vi "MultiAxisControl.vi"() -> ()   [LabVIEW 2026]
uses:
  Utility/AxisControl.ctl
  Parameters/GetAxisParameterString.vi
  Parameters/GetAxisParameterDouble.vi
  Motion/AbortSingle.vi
  Motion/MoveIncSingle.vi
  Motion/FreerunSingle.vi
  Motion/EnableSingle.vi
  Motion/DisableSingle.vi
  Motion/FaultAckSingle.vi
  Motion/HomeSingle.vi
panel:
  in  "Disconnect?":bool
  in  "Show First":i32=2 caption="Axes" min=0 max=32
  out "Status":string
  in  "StopProgram":bool caption="Stop"
  out "do stop":bool
  in  "stop":bool
  out "Error":string
  in  "Init":bool=TRUE
  in  "Abort Motion":bool
  in  "Reset Controller":bool
  in  "In Task:":i32(ring)=1 items=["TLibrary", "T01", "T02", "T03", "T04", "T05", "T06", "T07", "T08", "T09", "T10", "T11", "T12", "T13", "T14", "T15", "T16", "T17", "T18", "T19", "T20", "T21", "T22", "T23", "T24", "T25", "T26", "T27", "T28", "T29", "T30", "T31"]
  in  "ExecuteProgram":bool caption="Execute"
  in  "Program:":path
  in  "Axes":T1[](array[typedef])
  in  "Status":string
  in  "Execute":bool
  in  "Command:":string
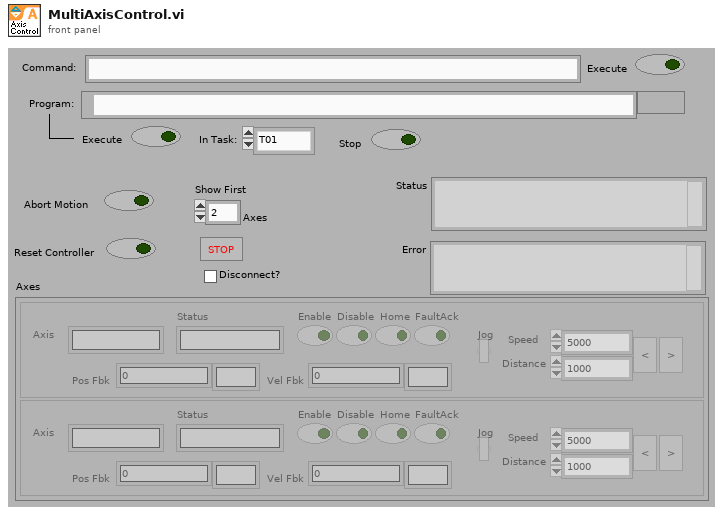
[diagram p1: front panel]
types:
  T1 = typedef "AxisControl.ctl" = cluster{"Axis":string, "Enable":bool, "Disable":bool, "Home":bool, "FaultAck":bool, "Jog":bool, "Speed":dbl, "Distance":dbl, "Jog Left":bool, "Jog Right":bool, "Status":string, "Pos Fbk":dbl, "Vel Fbk":dbl, "Pos Units":string, "Vel Units":string}
  T2 = cluster{"new reference":refnum<k24>, "Event Callback":refnum<k27>, "ControllerDiagPacket":refnum<user-event>, "Event Registration Refnum":refnum<event-registration>}
  T3 = enum32{"invalid app kind", "Development System", "Run Time System", "Student Edition", "Embedded LabVIEW", "Evaluation", "Custom"}
  T4 = cluster{"Axis":string, "Enable":bool, "Disable":bool, "Home":bool, "FaultAck":bool, "Jog":bool, "Speed":dbl, "Distance":dbl, "Jog Left":bool, "Jog Right":bool, "Status":string, "Pos Fbk":dbl, "Vel Fbk":dbl, "Pos Units":string, "Vel Units":string}
  T5 = typedef "AxisDiagPacket.ctl" = cluster{"Axis Name":string, "Analog Input 0":dbl, "Analog Input 1":dbl, "Axis Fault (num)":i32, "Axis Fault (str)":string, "Axis Fault (bits)":cluster{"AmplifierFault":bool, "AmplifierTemperatureFault":bool, "CcwEndOfTravelLimitFault":bool, "CcwSoftwareLimitFault":bool, "CommunicationLostFault":bool, "CwEndOfTravelLimitFault":bool, "CwSoftwareLimitFault":bool, "EmergencyStopFault":bool, "EncoderFault":bool, "ExternalFault":bool, "FeedbackScalingFault":bool, "GantryMisalignFault ":bool, "HallSensorFault":bool, "InPositionTimeoutFault":bool, "MarkerSearchFault":bool, "MaxVelocityCommandFault":bool, "MissedInterruptFault":bool, "MotorTemperatureFault":bool, "None":bool, "OverCurrentFault":bool, "PositionErrorFault":bool, "PositionFeedbackFault":bool, "PowerSupplyFault":bool, "ProbeInputFault":bool, "SafeZoneFault":bool, "VelocityErrorFault":bool, "VelocityFeedbackFault":bool, "VoltageClampFault":bool, "InternalFault":bool}, "Axis Status (num)":i32, "Axis Status (str)":string, "Axis Status (bits)":cluster{"BacklashActive":bool, "CalibrationEnabled1D":bool, "CalibrationEnabled2D":bool, "CommandValid":bool, "DriveAbortPending":bool, "DrivePending":bool, "Enabling":bool, "GainMappingEnabled":bool, "GantryAligned":bool, "GantryRealigning":bool, "Homed":bool, "Homing":bool, "IFOVEnabled":bool, "JogGenerating":bool, "Jogging":bool, "JoystickControl":bool, "MasterSlaveControl":bool, "MotionBlocked":bool, "MotionClamped":bool, "MoveDone":bool, "None":bool, "NotVirtual":bool, "Profiling":bool, "Stability0":bool, "Stability1":bool, "TrajectoryFiltering":bool, "WaitDone":bool}, "Current Command":sgl, "Current Error":sgl, "Current Feedback":sgl, "Digital Inputs":i32, "Digital Outputs":i32, "Drive Status":i32, "Drive Status (str)":string, "Drive Status (bits)":cluster{"AccelerationPhase":bool, "AutofocusActive":bool, "BrakeOutput":bool, "CcwEndOfTravelLimitInput":bool, "CosineEncoderError":bool, "CurrentClamp":bool, "CwEndOfTravelLimitInput":bool, "DecelerationPhase":bool, "DualLoopActive":bool, "EmergencyStopInput":bool, "Enabled":bool, "EncoderClipping":bool, "GalvoCalibrationEnabled":bool, "GalvoPowerCorrection":bool, "HallAInput":bool, "HallBInput":bool, "HallCInput":bool, "HighResolutionMode":bool, "HomeLimitInput":bool, "InPosition":bool, "InPosition2":bool, "MarkerInput":bool, "MarkerLatch":bool, "MoveActive":bool, "NoMotorSupply":bool, "None":bool, "PowerLimiting":bool, "ProgrammingFlash":bool, "ProgrammingMXH":bool, "PSOHaltLatch":bool, "ServoControl":bool, "SineEncoderError":bool}, "Position Feedback Auxiliary":dbl, "Position Command":dbl, "Position Error":dbl, "Position Feedback":dbl, "Program Position Command":dbl, "Program Position Error":dbl, "Program Position Feedback":dbl, "Velocity Command":dbl, "Velocity Error":dbl, "Velocity Feedback":dbl}
  T6 = cluster{"Axis":string, "Enable":bool, "Disable":bool, "Home":bool, "FaultAck":bool, "Jog":bool, "Speed":dbl, "Distance":dbl, "Jog Left":bool, "Jog Right":bool, "Status":string, "Pos Fbk":dbl, "Vel Fbk":dbl, "Pos Units":string, "Vel Units":string}[]
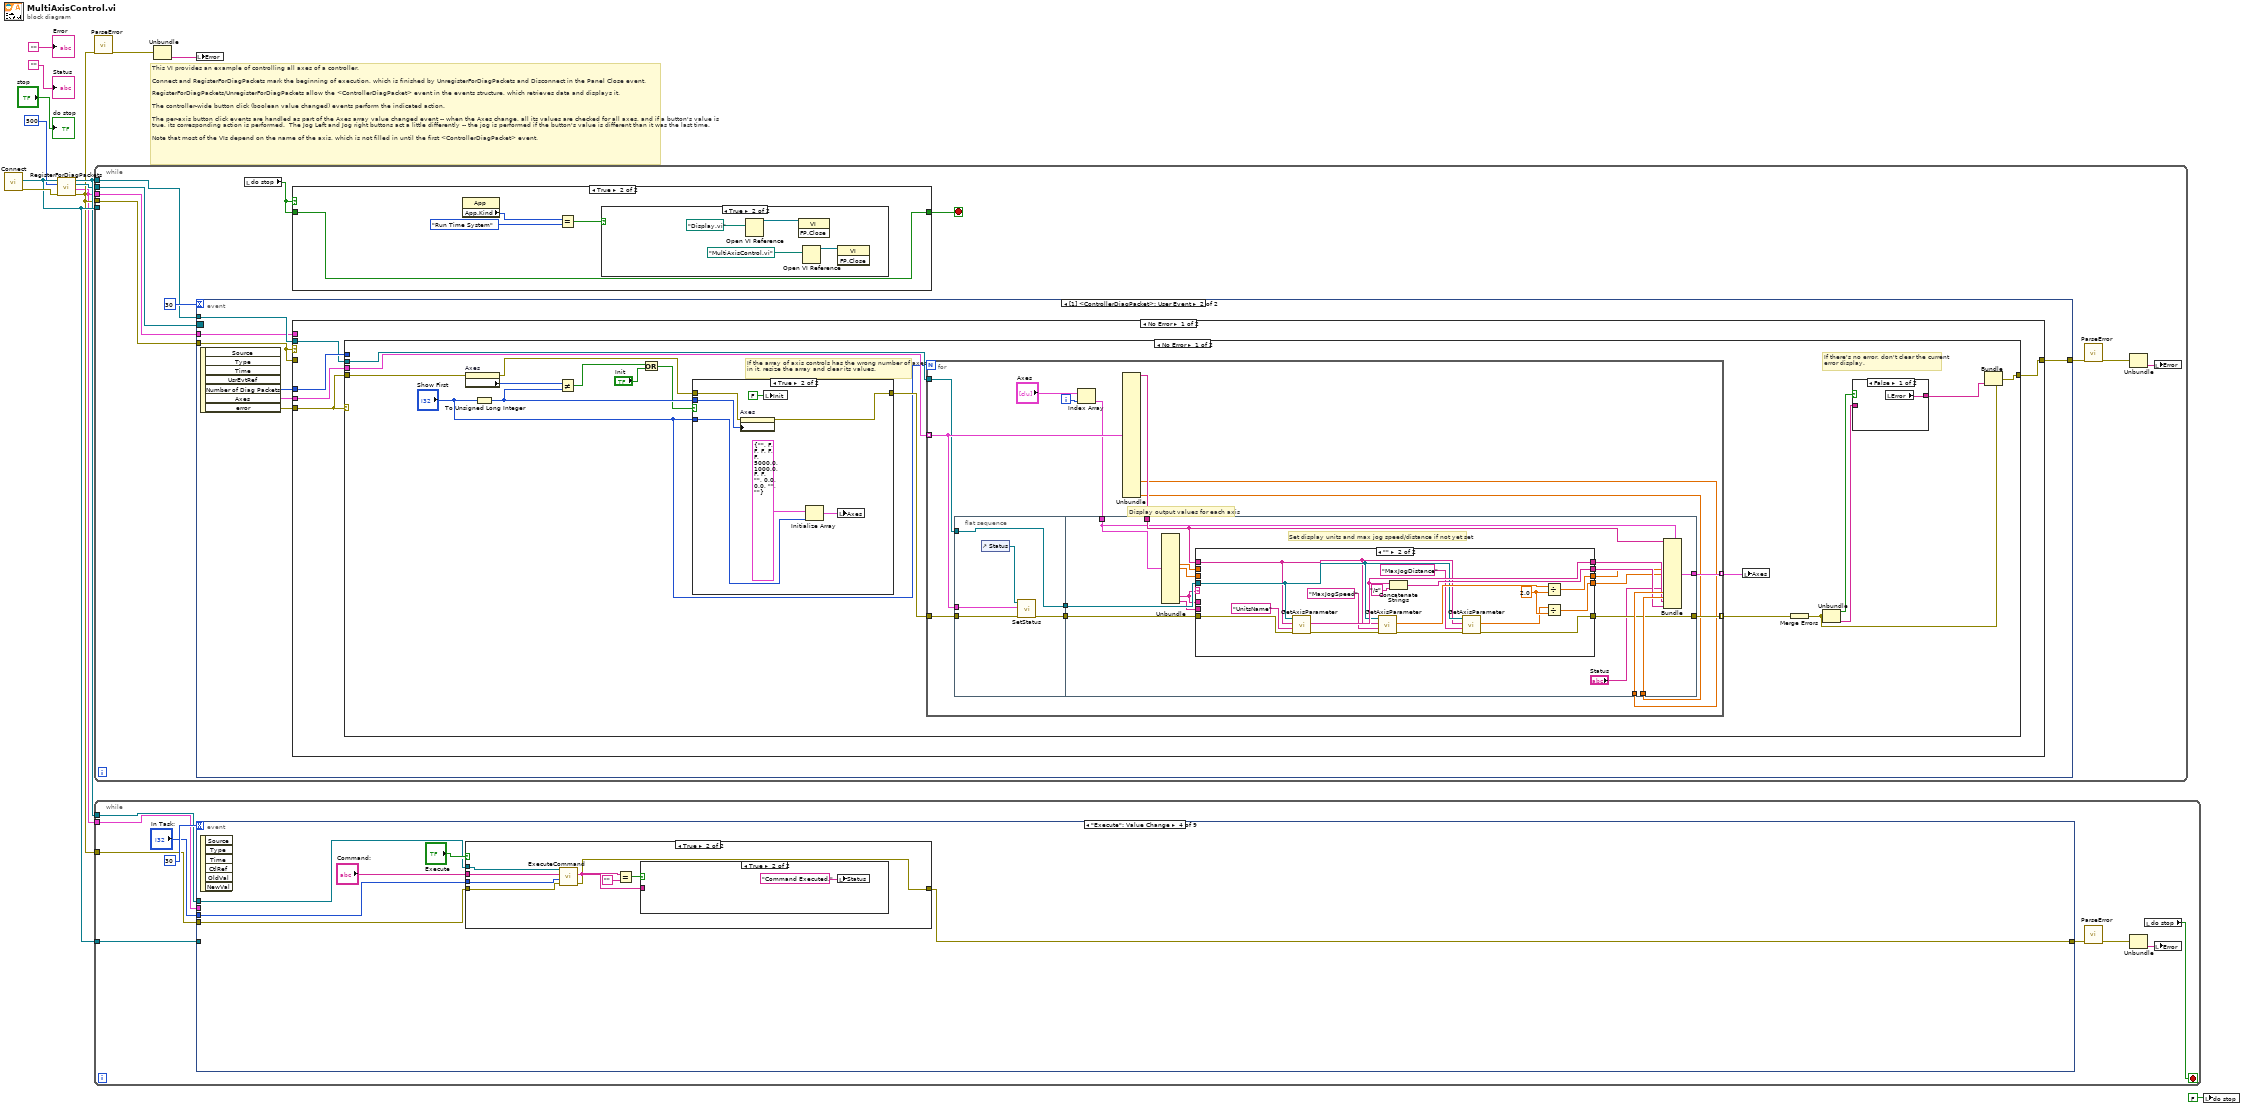
[diagram p0: block diagram]
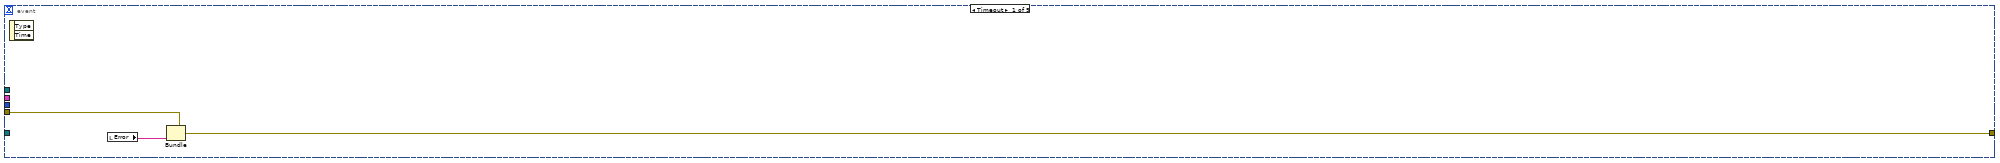
[diagram p2: hidden frame]
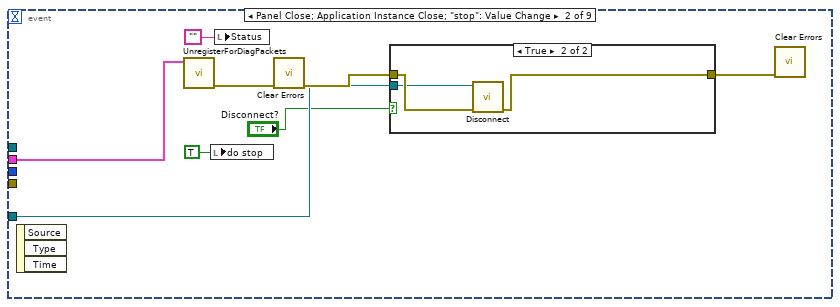
[diagram p3: hidden frame]
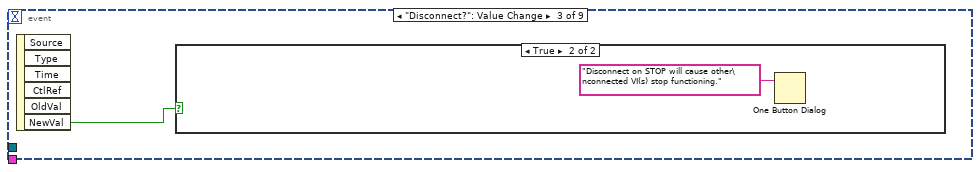
[diagram p5: hidden frame]
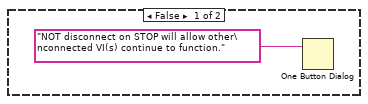
[diagram p6: hidden frame]
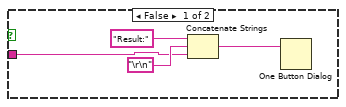
[diagram p8: hidden frame]
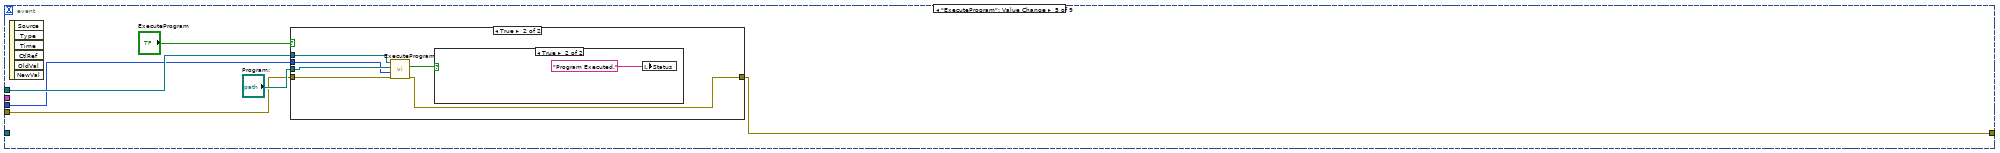
[diagram p9: hidden frame]
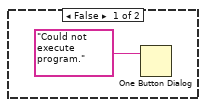
[diagram p11: hidden frame]
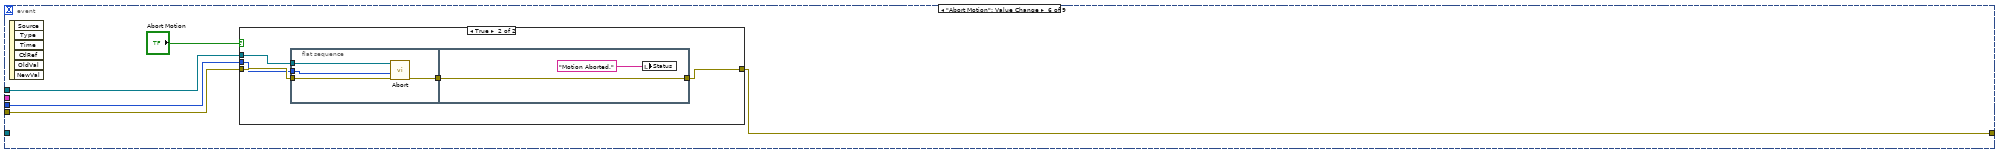
[diagram p12: hidden frame]
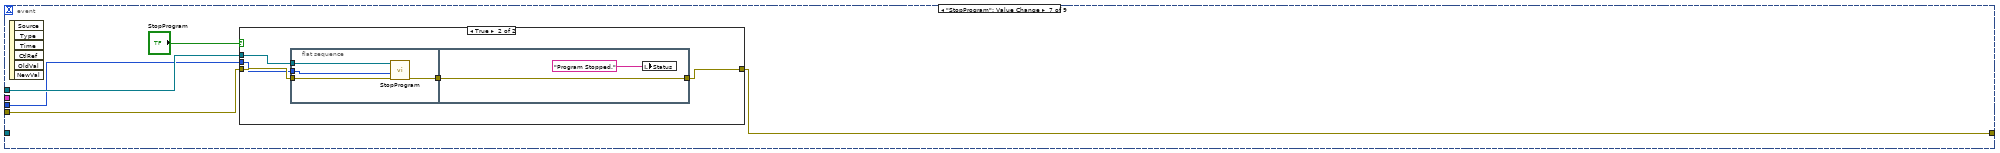
[diagram p14: hidden frame]
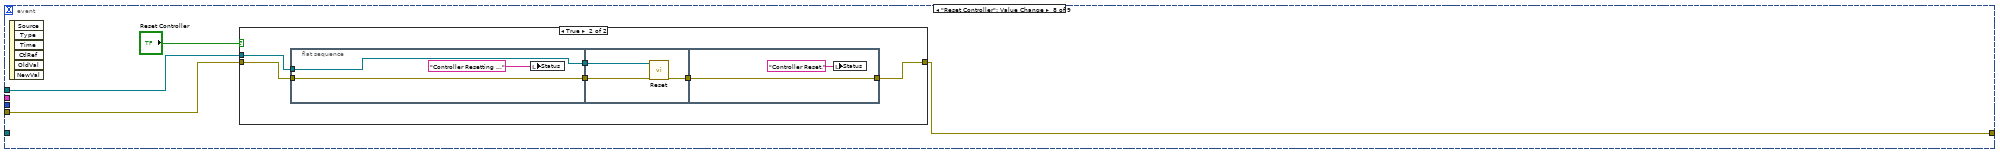
[diagram p16: hidden frame]
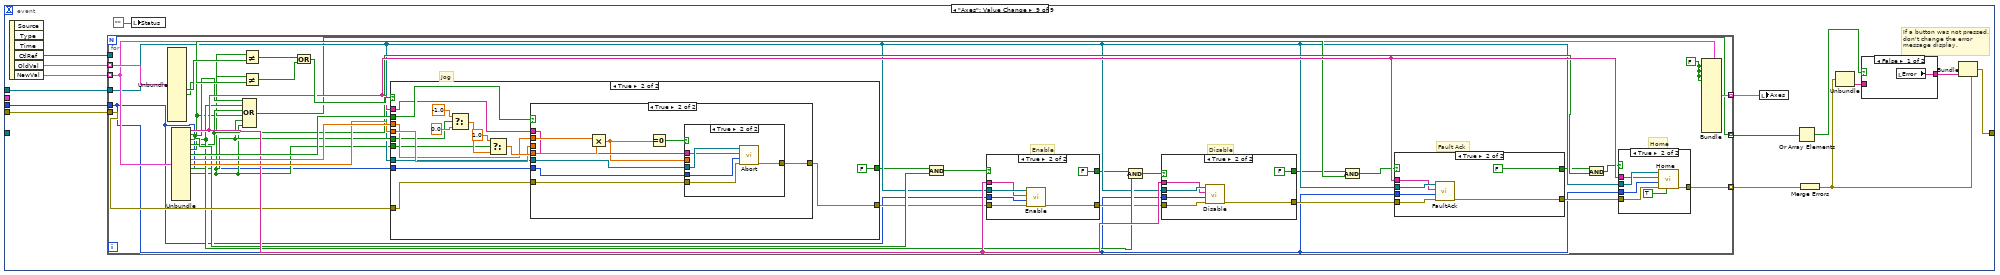
[diagram p18: hidden frame]
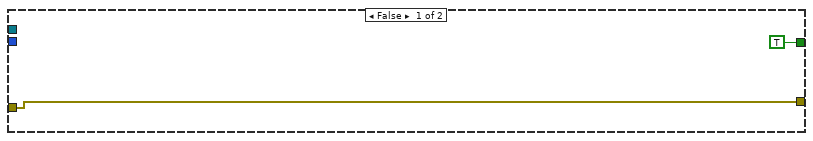
[diagram p20: hidden frame]
diagram:
  # "This VI provides an example of controlling all axes of a controller. \n\nConnect and RegisterForDiagPackets mark the beginning of execution, which is finished by UnregisterForDiagPackets and Disconnect in the Panel Close event.\n\nRegisterForDiagPackets/UnregisterForDiagPackets allow the <ControllerDiagPacket> event in the events structure, which retrieves data and displays it.\n\nThe controller-wide button click (boolean value changed) events perform the indicated action.\n\nThe per-axis button click events are handled as part of the Axes array value changed event -- when the Axes change, all its values are checked for all axes, and if a button's value is true, its corresponding action is performed.  The Jog Left and Jog right buttons act a little differently -- the jog is performed if the button's value is different than it was the last time.\n\nNote that most of the VIs depend on the name of the axis, which is not filled in until the first <ControllerDiagPacket> event."
  n1 = call "Connect.vi"() -> ("error out"=w7:errorcluster, "controller"=w6:refnum<k24>)  [unwired: 10 in]
  n2 = call "RegisterForDiagPackets.vi"("error in (no error)"=w7, "refresh interval (default)"=500, "Controller in"=w6) -> ("error out"=w3:errorcluster, "Event Metadata"=w2:T2, "Event Registration Refnum"=w4:refnum<event-registration>, "Controller out"=w5:refnum<k24>)  [unwired: 4 in]
  n3 = call "ParseError.vi"("error in (no error)"=w3) -> ("error out"=w11:errorcluster)  [unwired: 10 in]
  n4 = while {
    tunnel: w4 -> [w20]
    tunnel: w5 -> [w18]
    tunnel: w6 -> [_]
    tunnel: w3 -> [w17]
    tunnel: w2 -> [w16]
    stop <- w15 stop-if-true
    n5 = event shown="[1] <ControllerDiagPacket>: User Event" {
      selector: w20 -> [_ _]
      dyn-events: _ -> [_ _]
      timeout: 30 -> [_ _]
      tunnel: [w33 w42] -> w19
      tunnel: w18 -> [_ w41]
      tunnel: w17 -> [w35 w40]
      tunnel: w16 -> [_ w36]
      event Timeout {
        n6 = event-data() -> ()  [unwired: 1 in, 2 out]
        n7 = local read "Error"() -> (w34:string)
        n8 = Bundle(cluster=w35, "source"=w34) -> (w33:errorcluster)  [unwired: 2 in]
      }
      event User Event {
        n9 = event-data() -> ("Number of Diag Packets"=w39:i32, "Axes"=w38:T5[], "error"=w37:errorcluster)  [unwired: 1 in, 4 out]
        n10 = case shown="No Error" w40 {
          tunnel: w38 -> [w47 _]
          tunnel: [w46 w134] -> w42
          tunnel: w39 -> [w45 _]
          tunnel: w37 -> [w44 _]
          tunnel: w40 -> [_ w134]
          tunnel: w41 -> [w43 _]
          tunnel: w36 -> [_ _]
          frame No Error {
            n11 = case shown="No Error" w44 {
              tunnel: w47 -> [w65 _]
              tunnel: [w55 w133] -> w46
              tunnel: w44 -> [w51 w133]
              tunnel: w45 -> [_ _]
              tunnel: w43 -> [w49 _]
              frame No Error {
                # "If there's no error, don't clear the current error display."
                # "If the array of axis controls has the wrong number of axes in it, resize the array and clear its values."
                n12 = property on="Axes" class="Arr (strict)"(error in=w51) -> (error out=w50:errorcluster, "Number of Rows"=w61:u32)  [unwired: 1 in, 1 out]
                n13 = To Unsigned Long Integer(number="Show First") -> (unsigned 32bit integer=w60:u32)
                n14 = Not Equal?(x=w61, y=w60) -> (x != y?=w59:bool)
                n15 = Or(x=w59, y="Init") -> (x .or. y?=w58:bool)
                n16 = case shown="True" w58 {
                  tunnel: w50 -> [w125 w132]
                  tunnel: [w125 w131] -> w64
                  tunnel: w60 -> [_ w127]
                  tunnel: "Show First" -> [_ w128]
                  frame False {
                  }
                  frame True {
                    n17 = property on="Axes" class="Arr (strict)"(error in=w132, "Number of Rows"=w127) -> (error out=w131:errorcluster)  [unwired: 1 in, 1 out]
                    n18 = local write "Init"(FALSE ("Init")) -> ()
                    n19 = Initialize Array(T4 {"Axis"="", "Enable"=FALSE, "Disable"=FALSE, "Home"=FALSE, "FaultAck"=FALSE, "Jog"=FALSE, "Speed"=5000.0, "Distance"=1000.0, "Jog Left"=FALSE, "Jog Right"=FALSE, "Status"="", "Pos Fbk"=0.0, "Vel Fbk"=0.0, "Pos Units"="", "Vel Units"=""} ("Axis"), w128) -> (w130:T6)
                    n20 = local write "Axes"(w130) -> ()
                  }
                }
                n21 = for {
                  N: "Show First" -> [_]
                  tunnel: w64 -> [w79]
                  tunnel: w65 -> [w80] mode=indexing
                  tunnel: [w78] -> w63 mode=indexing
                  tunnel: [w73] -> w62 mode=indexing
                  tunnel: w49 -> [w71]
                  i -> [w74]
                  # "Display output values for each axis"
                  n22 = flat-sequence {
                    tunnel: w80 -> [w84]
                    tunnel: w79 -> [w83]
                    tunnel: [w82] -> w72
                    tunnel: w71 -> [w81]
                    tunnel: [w81] -> w70
                    tunnel: w75 -> [w95]
                    tunnel: w77 -> [w97]
                    tunnel: w69 -> [w101]
                    tunnel: w68 -> [w100]
                    tunnel: w72 -> [w98]
                    tunnel: w70 -> [w96]
                    tunnel: [w102] -> w78
                    tunnel: [w99] -> w73
                    frame #0 {
                      n23 = control-ref of="Status"() -> (w85:refnum<vi>)
                      n24 = call "SetStatus.vi"("error in (no error)"=w83, "AxisDiagPacket"=w84, "Status string"=w85) -> ("error out"=w82:errorcluster)  [unwired: 8 in]
                    }
                    frame #1 {
                      # "Set display units and max jog speed/distance if not yet set"
                      n25 = Unbundle(w95) -> ("Speed"=w90:dbl, "Distance"=w89:dbl, "Pos Units"=w94:string, "Vel Units"=w93:string)  [unwired: 11 out]
                      n26 = case shown="\"\"" w94 {
                        tunnel: w96 -> [_ w109]
                        tunnel: [w107 w112] -> w99
                        tunnel: w98 -> [w107 w122]
                        tunnel: w97 -> [_ w108]
                        tunnel: w94 -> [w105 _]
                        tunnel: w93 -> [w106 _]
                        tunnel: [w106 w121] -> w92
                        tunnel: [w105 w120] -> w91
                        tunnel: w90 -> [w104 _]
                        tunnel: w89 -> [w103 _]
                        tunnel: [w104 w111] -> w88
                        tunnel: [w103 w110] -> w87
                        frame Default {
                        }
                        frame "" {
                          w119 = 2.0 ("y")
                          n27 = call-poly "GetAxisParameter.vi"("error in (no error)"=w122, "Parameter Name"="UnitsName" ("parameter name"), "axis name"=w108, "controller in"=w109) -> ("error out"=w113:errorcluster, "value"=w120:string)  [unwired: 5 in, 1 out]
                          n28 = call-poly "GetAxisParameter.vi"("error in (no error)"=w113, "Parameter Name"="MaxJogSpeed" ("parameter name"), "axis name"=w108, "controller in"=w109) -> ("error out"=w114:errorcluster, "value"=w117:dbl)  [unwired: 5 in, 1 out]
                          n29 = Concatenate Strings(w120, "/s" ("string")) -> (w121:string)
                          n30 = call-poly "GetAxisParameter.vi"("error in (no error)"=w114, "Parameter Name"="MaxJogDistance" ("parameter name"), "axis name"=w108, "controller in"=w109) -> ("error out"=w112:errorcluster, "value"=w118:dbl)  [unwired: 5 in, 1 out]
                          n31 = Divide(x=w117, y=w119) -> (x/y=w111:dbl)
                          n32 = Divide(x=w118, y=w119) -> (x/y=w110:dbl)
                        }
                      }
                      n33 = Bundle(cluster=w95, "Axis"=w97, "Speed"=w88, "Distance"=w87, "Status"="Status", "Pos Fbk"=w101, "Vel Fbk"=w100, "Pos Units"=w91, "Vel Units"=w92) -> (w102:T1)  [unwired: 7 in]
                    }
                  }
                  n34 = Index Array(array="Axes", index=w74) -> (element=w75:T1)
                  n35 = Unbundle(w80) -> ("Axis Name"=w77:string, "Program Position Feedback"=w69:dbl, "Velocity Feedback"=w68:dbl)  [unwired: 24 out]
                }
                n36 = local write "Axes"(w63) -> ()
                n37 = Merge Errors(w62) -> (w56:errorcluster)
                n38 = Unbundle(w56) -> ("status"=w54:bool, "source"=w53:string)  [unwired: 1 out]
                n39 = case shown="False" w54 {
                  tunnel: w53 -> [_ w67]
                  tunnel: [w66 w67] -> w52
                  frame False {
                    n40 = local read "Error"() -> (w66:string)
                  }
                  frame True {
                  }
                }
                n41 = Bundle(cluster=w56, "source"=w52) -> (w55:errorcluster)  [unwired: 2 in]
              }
              frame Error {
              }
            }
          }
          frame Error {
          }
        }
      }
    }
    n42 = local read "do stop"() -> (w14:bool)
    n43 = case shown="True" w14 {
      tunnel: w14 -> [w24 w28]
      tunnel: [w24 w28] -> w15
      frame False {
      }
      frame True {
        n44 = property class="App"() -> ("App.Kind"=w27:T3)  [unwired: 2 in, 2 out]
        n45 = Equal?(x=w27, y=T3."Run Time System" ("Application:Kind")) -> (x = y?=w25:bool)
        n46 = case shown="True" w25 {
          frame False {
          }
          frame True {
            n47 = Open VI Reference(vi path=path "Display.vi") -> (vi reference=w29:refnum<vi>)  [unwired: 5 in, 1 out]
            n48 = invoke class="VI" method="FP.Close"(reference=w29) -> ()  [unwired: 2 in, 3 out]
            n49 = Open VI Reference(vi path=path "MultiAxisControl.vi") -> (vi reference=w31:refnum<vi>)  [unwired: 5 in, 1 out]
            n50 = invoke class="VI" method="FP.Close"(reference=w31) -> ()  [unwired: 2 in, 3 out]
          }
        }
      }
    }
    n51 = call "ParseError.vi"("error in (no error)"=w19) -> ("error out"=w22:errorcluster)  [unwired: 10 in]
    n52 = Unbundle(w22) -> ("source"=w23:string)  [unwired: 2 out]
    n53 = local write "Error"(w23) -> ()
  }
  n54 = while {
    tunnel: w6 -> [w140]
    tunnel: w5 -> [w139]
    tunnel: w3 -> [w138]
    tunnel: w2 -> [w135]
    stop <- w137 stop-if-true
    n55 = event shown="[3] \"Execute\": Value Change" {
      selector: _ -> [_ _ _ _ _ _ _ _ _]
      dyn-events: _ -> [_ _ _ _ _ _ _ _ _]
      timeout: 30 -> [_ _ _ _ _ _ _ _ _]
      tunnel: w139 -> [_ _ _ w167 w187 w201 w216 w234 w263]
      tunnel: w138 -> [w147 _ _ w166 w185 w202 w218 w233 w262]
      tunnel: [w146 _ _ w164 w184 w199 w217 w232 w257] -> w142
      tunnel: w140 -> [_ w154 _ _ _ _ _ _ _]
      tunnel: "In Task:" -> [_ _ _ w163 w183 w198 w215 _ w251]
      tunnel: w135 -> [_ w148 _ _ _ _ _ _ _]
      event Timeout {
        n56 = event-data() -> ()  [unwired: 1 in, 2 out]
        n57 = local read "Error"() -> (w145:string)
        n58 = Bundle(cluster=w147, "source"=w145) -> (w146:errorcluster)  [unwired: 2 in]
      }
      event Panel Close; Application Instance Close; "stop": Value Change {
        n59 = event-data() -> ()  [unwired: 1 in, 3 out]
        n60 = call "UnregisterForDiagPackets.vi"("Event Metadata"=w148) -> ("error out"=w149:errorcluster)  [unwired: 9 in]
        n61 = local write "do stop"(TRUE) -> ()
        n62 = local write "Status"("") -> ()
        n63 = call <vilib>:"Clear Errors.vi"("error in (no error)"=w149) -> ("error out"=w155:errorcluster)  [unwired: 5 in, 1 out]
        n64 = case shown="True" "Disconnect?" {
          tunnel: w155 -> [w156 w159]
          tunnel: w154 -> [_ w158]
          tunnel: [w156 w157] -> w153
          frame False {
          }
          frame True {
            n65 = call "Disconnect.vi"("error in (no error)"=w159, "controller"=w158) -> ("error out"=w157:errorcluster)  [unwired: 9 in]
          }
        }
        n66 = call <vilib>:"Clear Errors.vi"("error in (no error)"=w153) -> ()  [unwired: 5 in, 2 out]
      }
      event "Disconnect?": Value Change {
        n67 = event-data() -> ("NewVal"=w160:bool)  [unwired: 1 in, 5 out]
        n68 = case shown="True" w160 {
          frame False {
            n69 = One Button Dialog(message="NOT disconnect on STOP will allow other\nconnected VI(s) continue to function.") -> ()  [unwired: 1 in, 1 out]
          }
          frame True {
            n70 = One Button Dialog(message="Disconnect on STOP will cause other\nconnected VI(s) stop functioning.") -> ()  [unwired: 1 in, 1 out]
          }
        }
      }
      event "Execute": Value Change {
        n71 = event-data() -> ()  [unwired: 1 in, 6 out]
        n72 = case shown="True" "Execute" {
          tunnel: w167 -> [_ w177]
          tunnel: w166 -> [w169 w175]
          tunnel: "Command:" -> [_ w176]
          tunnel: [w169 w171] -> w164
          tunnel: w163 -> [_ w170]
          frame False {
          }
          frame True {
            n73 = call "ExecuteCommand.vi"("error in (no error)"=w175, "taskId"=w170, "Command Code"=w176, "controller in"=w177) -> ("error out"=w171:errorcluster, "return value"=w172:string)  [unwired: 5 in, 1 out]
            n74 = Equal?(x=w172, y="") -> (x = y?=w173:bool)
            n75 = case shown="True" w173 {
              tunnel: w172 -> [w178 _]
              frame False {
                n76 = Concatenate Strings("Result:", "\r\n", w178) -> (w181:string)
                n77 = One Button Dialog(message=w181) -> ()  [unwired: 1 in, 1 out]
              }
              frame True {
                n78 = local write "Status"("Command Executed." ("Status")) -> ()
              }
            }
          }
        }
      }
      event "ExecuteProgram": Value Change {
        n79 = event-data() -> ()  [unwired: 1 in, 6 out]
        n80 = case shown="True" "ExecuteProgram" {
          tunnel: w187 -> [_ w195]
          tunnel: w185 -> [w189 w193]
          tunnel: "Program:" -> [_ w194]
          tunnel: w183 -> [_ w191]
          tunnel: [w189 w190] -> w184
          frame False {
          }
          frame True {
            n81 = call "ExecuteProgram.vi"("error in (no error)"=w193, "taskId"=w191, "program name and path"=w194, "controller in"=w195) -> ("error out"=w190:errorcluster, "success"=w192:bool)  [unwired: 5 in, 1 out]
            n82 = case shown="True" w192 {
              frame False {
                n83 = One Button Dialog(message="Could not execute program.") -> ()  [unwired: 1 in, 1 out]
              }
              frame True {
                n84 = local write "Status"("Program Executed." ("Status")) -> ()
              }
            }
          }
        }
      }
      event "Abort Motion": Value Change {
        n85 = event-data() -> ()  [unwired: 1 in, 6 out]
        n86 = case shown="True" "Abort Motion" {
          tunnel: w201 -> [_ w208]
          tunnel: w202 -> [w203 w207]
          tunnel: [w203 w206] -> w199
          tunnel: w198 -> [_ w204]
          frame False {
          }
          frame True {
            n87 = flat-sequence {
              tunnel: w208 -> [w212]
              tunnel: w207 -> [w211]
              tunnel: [w210] -> w205
              tunnel: w204 -> [w209]
              tunnel: [w214] -> w206
              tunnel: w205 -> [w214]
              frame #0 {
                n88 = call-poly "Abort.vi"("error in (no error)"=w211, "taskId"=w209, "controller in"=w212) -> ("error out"=w210:errorcluster)  [unwired: 7 in, 1 out]
              }
              frame #1 {
                n89 = local write "Status"("Motion Aborted." ("Status")) -> ()
              }
            }
          }
        }
      }
      event "StopProgram": Value Change {
        n90 = event-data() -> ()  [unwired: 1 in, 6 out]
        n91 = case shown="True" "StopProgram" {
          tunnel: w218 -> [w220 w225]
          tunnel: [w220 w224] -> w217
          tunnel: w216 -> [_ w223]
          tunnel: w215 -> [_ w221]
          frame False {
          }
          frame True {
            n92 = flat-sequence {
              tunnel: w225 -> [w229]
              tunnel: w223 -> [w227]
              tunnel: [w228] -> w222
              tunnel: w221 -> [w226]
              tunnel: [w231] -> w224
              tunnel: w222 -> [w231]
              frame #0 {
                n93 = call "StopProgram.vi"("error in (no error)"=w229, "taskId"=w226, "controller in"=w227) -> ("error out"=w228:errorcluster)  [unwired: 7 in, 1 out]
              }
              frame #1 {
                n94 = local write "Status"("Program Stopped." ("Status")) -> ()
              }
            }
          }
        }
      }
      event "Reset Controller": Value Change {
        n95 = event-data() -> ()  [unwired: 1 in, 6 out]
        n96 = case shown="True" "Reset Controller" {
          tunnel: w234 -> [_ w242]
          tunnel: w233 -> [w236 w241]
          tunnel: [w236 w240] -> w232
          frame False {
          }
          frame True {
            n97 = flat-sequence {
              tunnel: w241 -> [w244]
              tunnel: w242 -> [w245]
              tunnel: [w245] -> w239
              tunnel: [w244] -> w238
              tunnel: w239 -> [w248]
              tunnel: w238 -> [w247]
              tunnel: [w246] -> w237
              tunnel: [w250] -> w240
              tunnel: w237 -> [w250]
              frame #0 {
                n98 = local write "Status"("Controller Resetting ..." ("Errors")) -> ()
              }
              frame #1 {
                n99 = call "Reset.vi"("error in (no error)"=w247, "controller in"=w248) -> ("error out"=w246:errorcluster)  [unwired: 8 in, 1 out]
              }
              frame #2 {
                n100 = local write "Status"("Controller Reset." ("Status")) -> ()
              }
            }
          }
        }
      }
      event "Axes": Value Change {
        # "If a button was not pressed, don't change the error message display."
        n101 = event-data() -> ("CtlRef"=w264:refnum<vi>, "OldVal"=w261:T1[], "NewVal"=w265:T1[])  [unwired: 1 in, 3 out]
        n102 = for {
          tunnel: w265 -> [w287] mode=indexing
          tunnel: w264 -> [_]
          tunnel: w263 -> [w285]
          tunnel: w262 -> [w293]
          tunnel: w261 -> [w300] mode=indexing
          tunnel: [w274] -> w260 mode=indexing
          tunnel: [w270] -> w259 mode=indexing
          tunnel: [w288] -> w254 mode=indexing
          tunnel: w251 -> [w268]
          w269 = FALSE
          # "Jog"
          # "Fault Ack"
          # "Home"
          # "Disable"
          # "Enable"
          n103 = Unbundle(w300) -> ("Jog Left"=w296:bool, "Jog Right"=w295:bool)  [unwired: 13 out]
          n104 = Unbundle(w287) -> ("Axis"=w294:string, "Enable"=w292:bool, "Disable"=w291:bool, "Home"=w290:bool, "FaultAck"=w289:bool, "Jog"=w301:bool, "Speed"=w303:dbl, "Distance"=w302:dbl, "Jog Left"=w286:bool, "Jog Right"=w275:bool)  [unwired: 5 out]
          n105 = Compound Arithmetic op=OR(w292, w291, w290, w289, w286, w275) -> (w270:bool)
          n106 = Not Equal?(x=w275, y=w296) -> (x != y?=w298:bool)
          n107 = Not Equal?(x=w286, y=w295) -> (x != y?=w297:bool)
          n108 = Or(x=w298, y=w297) -> (x .or. y?=w299:bool)
          n109 = case shown="True" w299 {
            tunnel: w301 -> [_ w316]
            tunnel: w303 -> [_ w314]
            tunnel: w302 -> [_ w315]
            tunnel: w275 -> [_ w310]
            tunnel: w286 -> [_ w309]
            tunnel: w285 -> [_ w313]
            tunnel: w294 -> [_ w312]
            tunnel: w293 -> [w305 w311]
            tunnel: [w305 w308] -> w278
            tunnel: [TRUE FALSE] -> w283
            tunnel: w268 -> [_ w306]
            frame False {
            }
            frame True {
              n110 = Select(t=-1.0, s=w309, f=0.0) -> (s? t:f=w321:dbl)
              n111 = Select(t=1.0, s=w310, f=w321) -> (s? t:f=w317:dbl)
              n112 = case shown="True" w316 {
                tunnel: w314 -> [w325 w339]
                tunnel: w315 -> [w330 _]
                tunnel: w317 -> [w329 w338]
                tunnel: w311 -> [w328 w337]
                tunnel: w312 -> [w324 w336]
                tunnel: w313 -> [w323 w335]
                tunnel: [w327 w334] -> w308
                tunnel: w306 -> [w322 w333]
                frame False {
                  n113 = Multiply(x=w330, y=w329) -> (x*y=w326:dbl)
                  n114 = call-poly "MoveInc.vi"("distance"=w326, "speed"=w325, "error in (no error)"=w328, "taskId"=w322, "axis name"=w324, "controller in"=w323) -> ("error out"=w327:errorcluster)  [unwired: 4 in, 1 out]
                }
                frame True {
                  n115 = Multiply(x=w339, y=w338) -> (x*y=w331:dbl)
                  n116 = Equal To 0?(x=w331) -> (x = 0?=w332:bool)
                  n117 = case shown="True" w332 {
                    tunnel: w337 -> [w345 w350]
                    tunnel: w336 -> [w344 w347]
                    tunnel: w335 -> [w343 w348]
                    tunnel: [w342 w349] -> w334
                    tunnel: w331 -> [w341 _]
                    tunnel: w333 -> [w340 w346]
                    frame False {
                      n118 = call-poly "Freerun.vi"("speed"=w341, "error in (no error)"=w345, "taskId"=w340, "axis name"=w344, "controller in"=w343) -> ("error out"=w342:errorcluster)  [unwired: 5 in, 1 out]
                    }
                    frame True {
                      n119 = call-poly "Abort.vi"("error in (no error)"=w350, "taskId"=w346, "axis name? (all)"=w347, "controller in"=w348) -> ("error out"=w349:errorcluster)  [unwired: 6 in, 1 out]
                    }
                  }
                }
              }
            }
          }
          n120 = And(x=w283, y=w292) -> (x .and. y?=w284:bool)
          n121 = case shown="True" w284 {
            tunnel: w285 -> [_ w381]
            tunnel: w278 -> [w375 w380]
            tunnel: w294 -> [_ w378]
            tunnel: [w375 w379] -> w277
            tunnel: [TRUE FALSE] -> w281
            tunnel: w268 -> [_ w376]
            frame False {
            }
            frame True {
              n122 = call-poly "Enable.vi"("error in (no error)"=w380, "taskId"=w376, "axis name"=w378, "controller in"=w381) -> ("error out"=w379:errorcluster)  [unwired: 6 in, 1 out]
            }
          }
          n123 = And(x=w281, y=w291) -> (x .and. y?=w282:bool)
          n124 = case shown="True" w282 {
            tunnel: w285 -> [_ w373]
            tunnel: w277 -> [w367 w371]
            tunnel: w294 -> [_ w372]
            tunnel: [w367 w370] -> w276
            tunnel: [TRUE FALSE] -> w279
            tunnel: w268 -> [_ w368]
            frame False {
            }
            frame True {
              n125 = call-poly "Disable.vi"("error in (no error)"=w371, "taskId"=w368, "axis name"=w372, "controller in"=w373) -> ("error out"=w370:errorcluster)  [unwired: 6 in, 1 out]
            }
          }
          n126 = And(x=w279, y=w289) -> (x .and. y?=w280:bool)
          n127 = case shown="True" w280 {
            tunnel: w285 -> [_ w358]
            tunnel: w276 -> [w352 w356]
            tunnel: w294 -> [_ w357]
            tunnel: [w352 w355] -> w273
            tunnel: [TRUE FALSE] -> w271
            tunnel: w268 -> [_ w353]
            frame False {
            }
            frame True {
              n128 = call-poly "FaultAck.vi"("error in (no error)"=w356, "taskId"=w353, "axis name"=w357, "controller in"=w358) -> ("error out"=w355:errorcluster)  [unwired: 6 in, 1 out]
            }
          }
          n129 = And(x=w271, y=w290) -> (x .and. y?=w272:bool)
          n130 = case shown="True" w272 {
            tunnel: w285 -> [_ w365]
            tunnel: w294 -> [_ w364]
            tunnel: w273 -> [w359 w363]
            tunnel: [w359 w362] -> w274
            tunnel: w268 -> [_ w360]
            frame False {
            }
            frame True {
              n131 = call-poly "Home.vi"("return immediately"=TRUE ("Return Immediately ?"), "error in (no error)"=w363, "taskId"=w360, "axis name"=w364, "controller in"=w365) -> ("error out"=w362:errorcluster)  [unwired: 5 in, 1 out]
            }
          }
          n132 = Bundle(cluster=w287, "Enable"=w269, "Disable"=w269, "Home"=w269, "FaultAck"=w269) -> (w288:T1)  [unwired: 11 in]
        }
        n133 = local write "Status"("") -> ()
        n134 = local write "Axes"(w254) -> ()
        n135 = Or Array Elements(Boolean array=w259) -> (logical OR=w258:bool)
        n136 = Merge Errors(w260) -> (w253:errorcluster)
        n137 = Unbundle(w253) -> ("source"=w256:string)  [unwired: 2 out]
        n138 = case shown="False" w258 {
          tunnel: w256 -> [_ w267]
          tunnel: [w266 w267] -> w255
          frame False {
            n139 = local read "Error"() -> (w266:string)
          }
          frame True {
          }
        }
        n140 = Bundle(cluster=w253, "source"=w255) -> (w257:errorcluster)  [unwired: 2 in]
      }
    }
    n141 = call "ParseError.vi"("error in (no error)"=w142) -> ("error out"=w144:errorcluster)  [unwired: 10 in]
    n142 = Unbundle(w144) -> ("source"=w143:string)  [unwired: 2 out]
    n143 = local read "do stop"() -> (w137:bool)
    n144 = local write "Error"(w143) -> ()
  }
  n145 = Unbundle(w11) -> ("source"=w12:string)  [unwired: 2 out]
  n146 = local write "Error"(w12) -> ()
  n147 = local write "do stop"(FALSE ("do stop")) -> ()
  "Error" <- ""
  "do stop" <- "stop"
  "Status" <- ""
